vi "FPGA_small2-2.vi"() -> ()   [LabVIEW 2018]
uses:
  <vilib>/Platform/TimedLoop/XDataNode/timing_clust.ctl
  <vilib>/Platform/TimedLoop/XDataNode/nitl_modes.ctl
  <vilib>/Platform/TimedLoop/XDataNode/wakeup.ctl
  <vilib>/rvi/Emulation/niFpgaGetClockAttributes.vi
  <vilib>/rvi/Emulation/niFpgaSctlEmulationGetInTimedLoop.vi
  <vilib>/rvi/Emulation/niFpgaEmulationReportErrorSimple.vi
  <vilib>/rvi/eio/common/nirviEmuTemplateMethod_errors.vi
  <vilib>/rvi/Emulation/niFpgaCriticalErrorInLSC.vi
  <vilib>/rvi/Emulation/niFpgaProcessEmulError.vi
  <vilib>/eio/EIONode/EIONode.xnode
  <vilib>/platform/TimedLoop/XDataNode/XDataNode.xnode
  <vilib>/Platform/TimedLoop/XDataNode/XDNodeRunTimeDep.lvlib
panel:
  in  "speed_scale":i16=1500
  out "speed":i16
  in  "offtrack limit":i16=1500
  out "AI0":u16=1344
  out "dAI":i16=8
  in  "delay ai ms":u32=1
  in  "pwm_val":u32=100
  in  "dt_pwm_us":u32=30 caption="Count(uSec)"
  out "busy":bool
  in  "dt_ctrl_us":u32=1 caption="delay_M_ms"
  in  "set_point":i16
  in  "stop_band":i16=4
  in  "inv":bool=TRUE
  out "gap_pos":i16=-1
  out "backward":bool
  out "position":i16=1241
  out "err cnt":i16
  in  "reset":bool
  out "off_track":bool
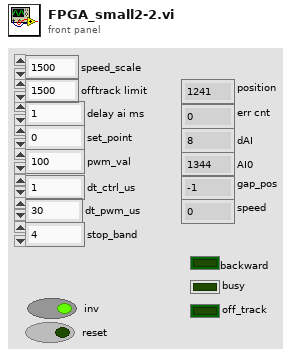
[diagram p1: front panel]
types:
  T1 = typedef "XDNodeRunTimeDep.lvlib/timing_clust.ctl" = cluster{"Expected End [f-1]":u64, "Actual End [f-1]":u64, "Finished Late? [f-1]":bool, "Expected End [i-1]":u64, "Actual End [i-1]":u64, "Finished Late? [i-1]":bool, "Expected Start [i]":u64, "Actual Start [i]":u64, "Expected Start [f]":u64, "Actual Start [f]":u64, "Source Name":string, "Structure Name":string, "Period":i64, "Deadline":i64, "Offset":i64, "Start":i64, "Priority":i32, "Timeout":i32, "Mode":T2, "Wakeup Reason":T3, "Error":errorcluster, "Source Type":string, "Secondary Source Type":string, "Global End Time":u64, "Global Start Time":u64, "Frame Duration":u64, "Iteration Duration":u64, "Assigned CPU":i32, "I/O Scan Engine Mode":u32}
  T2 = typedef "XDNodeRunTimeDep.lvlib/nitl_modes.ctl" = enum32{"No Change", "Process missed periods, maintain original phase", "Discard missed periods, maintain original phase", "Process missed periods, ignore original phase", "Discard missed periods, ignore original phase"}
  T3 = typedef "XDNodeRunTimeDep.lvlib/wakeup.ctl" = enum32{"Normal", "Aborted", "Asynchronous wakeup", "Timing source error", "Timed loop error", "Timeout"}
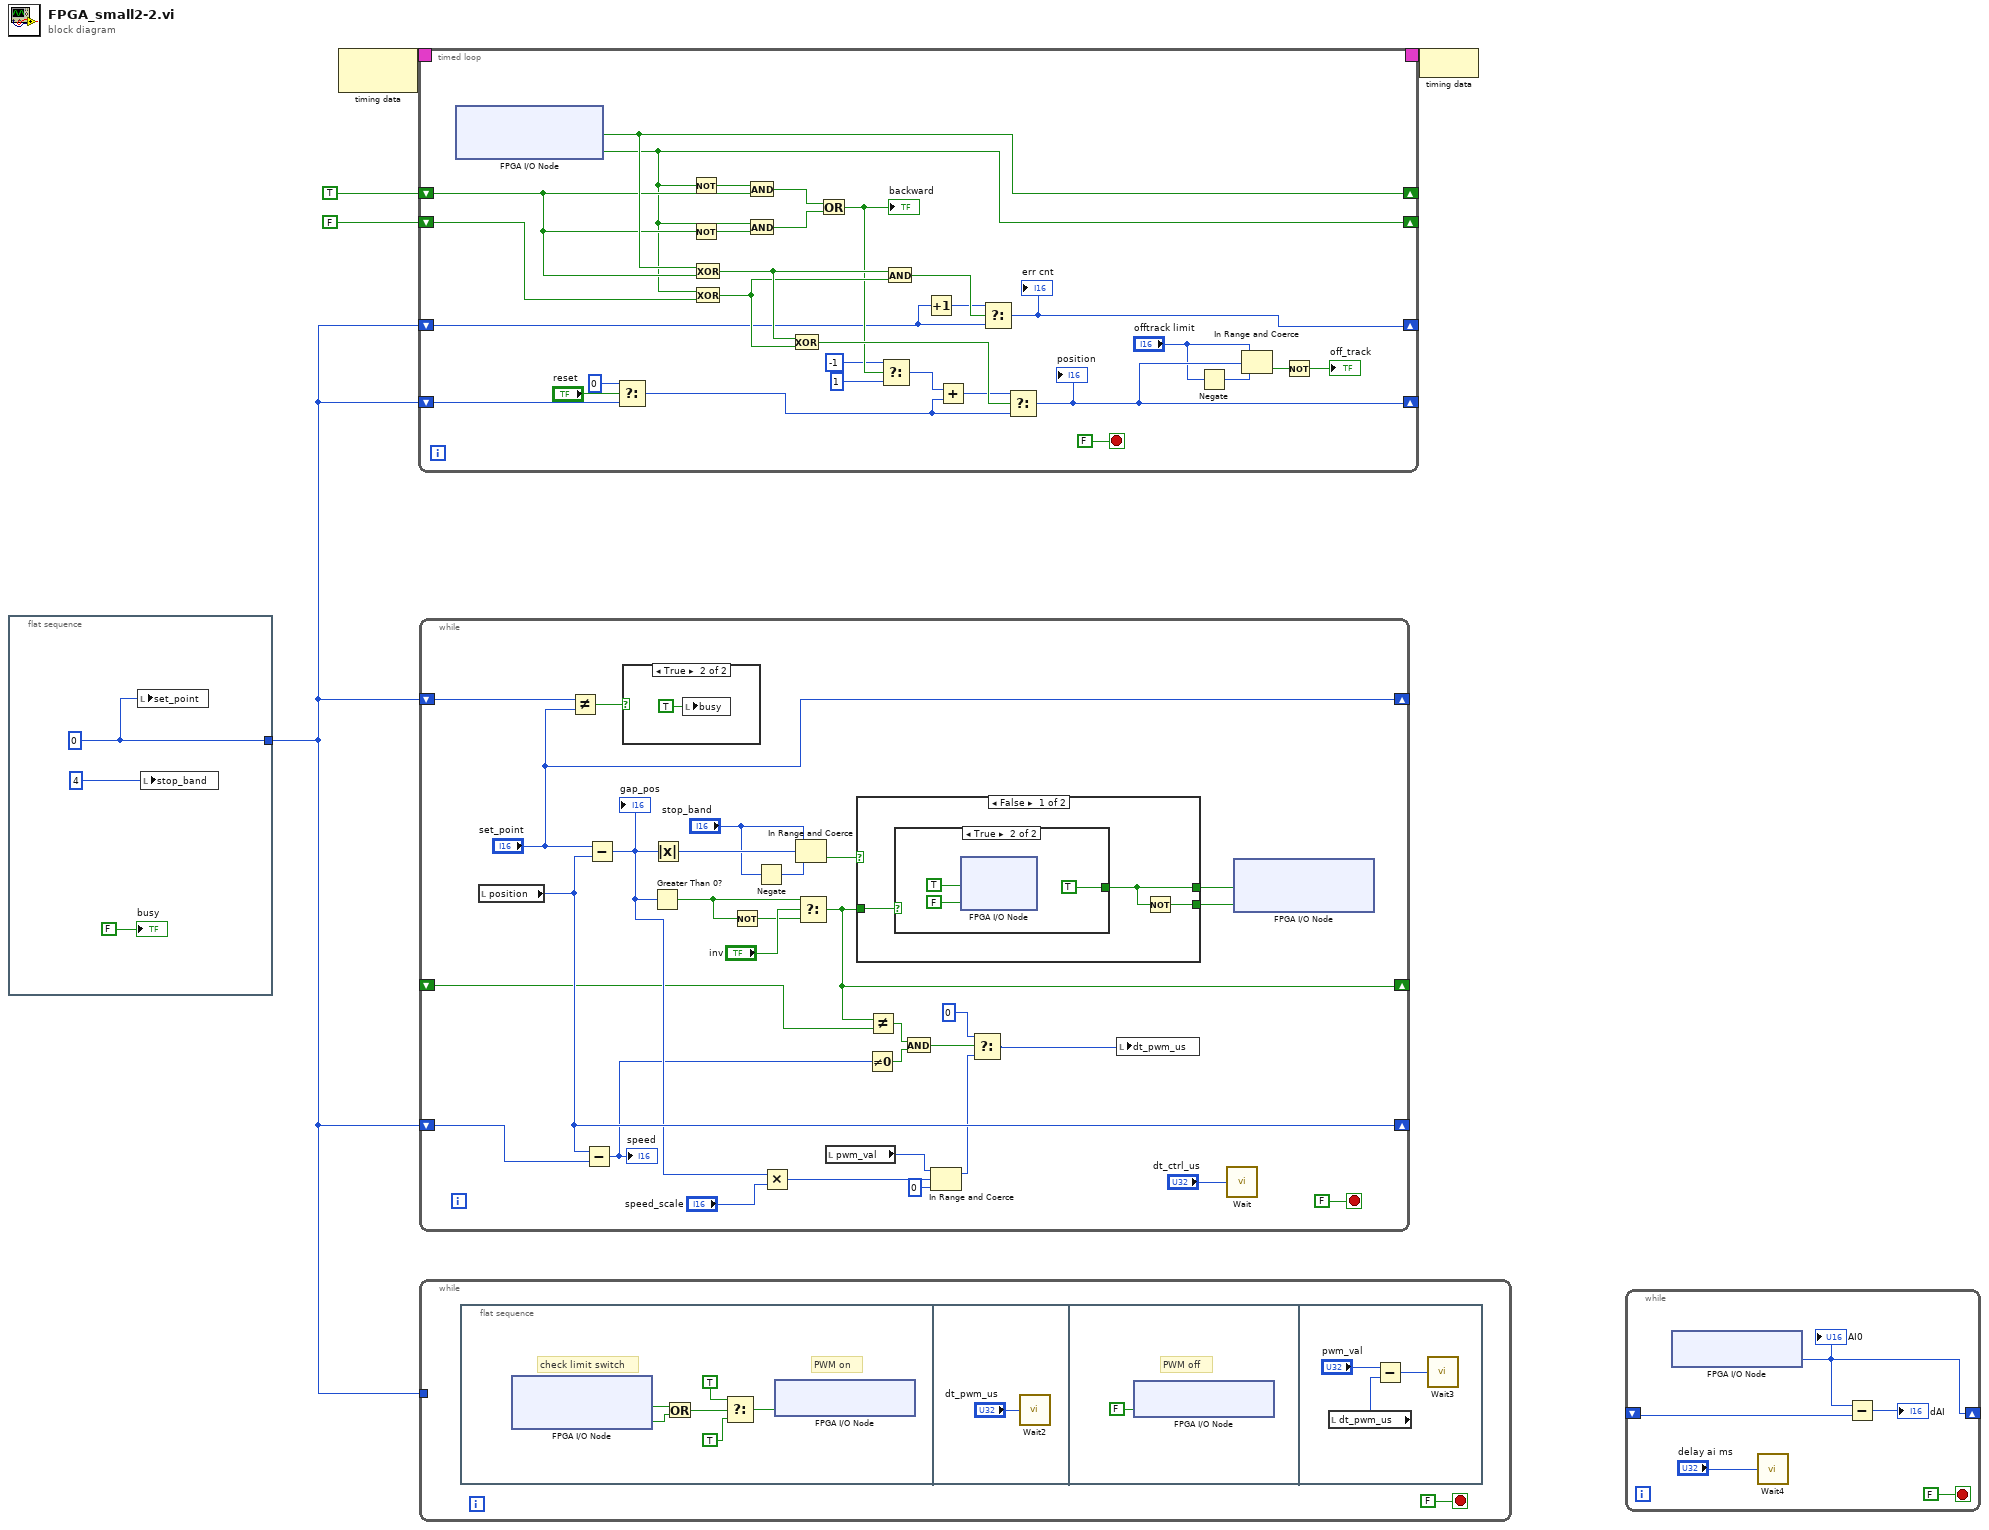
[diagram p0: block diagram]
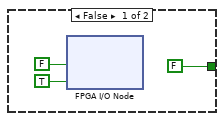
[diagram p3: hidden frame]
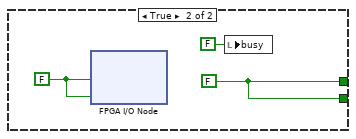
[diagram p4: hidden frame]
diagram:
  n1 = flat-sequence {
    tunnel: [w7] -> w1
    frame #0 {
      w7 = i16 0
      n2 = local write "set_point"(w7) -> ()
      n3 = local write "stop_band"(i16 4 ("dead band")) -> ()
      "busy" <- FALSE ("status")
    }
  }
  n4 = node-c288() -> (w5:T1)  [unwired: 1 in]
  n5 = timed-loop {
    timing: w5 -> [_]
    timing-out: [_] -> w4
    shift-right: [w33] -> _
    shift-left: TRUE ("ConnectorA/DIO11") -> [w32]
    shift-right: [w31] -> _
    shift-left: FALSE ("ConnectorA/DIO12") -> [w30]
    shift-right: [w13] -> _
    shift-left: w1 -> [w16]
    shift-right: [w18] -> _
    shift-left: w1 -> [w19]
    stop <- FALSE stop-if-true
    n6 = xnode "FPGA I/O Node"() -> ("ConnectorA/DIO11"=w33:bool, "ConnectorA/DIO12"=w31:bool)  [unwired: 2 in, 2 out]
    n7 = Select(t=i16 0, s="reset", f=w16) -> (s? t:f=w14:i16)
    n8 = Not(x=w31) -> (.not. x?=w37:bool)
    n9 = Not(x=w32) -> (.not. x?=w36:bool)
    n10 = Exclusive Or(1:w32, 2:w33) -> (0:w29:bool)
    n11 = Exclusive Or(1:w30, 2:w31) -> (0:w28:bool)
    n12 = And(x=w37, y=w32) -> (x .and. y?=w34:bool)
    n13 = And(x=w31, y=w36) -> (x .and. y?=w35:bool)
    n14 = Exclusive Or(1:w28, 2:w29) -> (0:w27:bool)
    n15 = Or(x=w34, y=w35) -> (x .or. y?=w26:bool)
    "backward" <- w26
    n16 = Select(t=i16 -1, s=w26, f=i16 1) -> (s? t:f=w23:i16)
    n17 = And(x=w29, y=w28) -> (x .and. y?=w21:bool)
    n18 = Increment(x=w19) -> (x+1=w20:i16)
    n19 = Add(x=w23, y=w14) -> (x+y=w22:i16)
    n20 = Select(t=w20, s=w21, f=w19) -> (s? t:f=w18:i16)
    "err cnt" <- w18
    n21 = Select(t=w22, s=w27, f=w14) -> (s? t:f=w13:i16)
    "position" <- w13
    n22 = Negate(x="offtrack limit") -> (-x=w10:i16)
    n23 = In Range and Coerce(upper limit="offtrack limit", x=w13, lower limit=w10) -> (In Range?=w12:bool)  [unwired: 1 out]
    n24 = Not(x=w12) -> (.not. x?=→"off_track":bool)
  }
  n25 = while {
    shift-right: ["set_point"] -> _
    shift-left: w1 -> [w58]
    shift-right: [w56] -> _
    shift-left: w1 -> [w55]
    shift-right: [w49] -> _
    shift-left: _ -> [w48]
    stop <- FALSE stop-if-true
    n26 = local read "position"() -> (w56:i16)
    n27 = Not Equal?(x=w58, y="set_point") -> (x != y?=w57:bool)
    n28 = Subtract(x=w56, y=w55) -> (x-y=w47:i16)
    "speed" <- w47
    n29 = Subtract(x="set_point", y=w56) -> (x-y=w53:i16)
    "gap_pos" <- w53
    n30 = case shown="True" w57 {
      frame False {
      }
      frame True {
        n31 = local write "busy"(TRUE ("busy")) -> ()
      }
    }
    n32 = Greater Than 0?(x=w53) -> (x > 0?=w60:bool)
    n33 = Absolute Value(x=w53) -> (abs(x)=w66:i16)
    n34 = Not(x=w60) -> (.not. x?=w61:bool)
    n35 = Negate(x="stop_band") -> (-x=w65:i16)
    n36 = Multiply(x=w53, y="speed_scale") -> (x*y=w52:i16)
    n37 = In Range and Coerce(upper limit="stop_band", x=w66, lower limit=w65) -> (In Range?=w63:bool)  [unwired: 1 out]
    n38 = Select(t=w60, s="inv", f=w61) -> (s? t:f=w49:bool)
    n39 = local read "pwm_val"() -> (w51:u32)
    n40 = case shown="False" w63 {
      tunnel: [w74 w83] -> w68
      tunnel: [w73 w83] -> w67
      tunnel: w49 -> [w72 _]
      frame False {
        n41 = case shown="True" w72 {
          tunnel: [FALSE ("dir") TRUE ("dir")] -> w73
          frame False {
            n42 = xnode "FPGA I/O Node"("LED0"=FALSE, "LED1"=TRUE) -> ()  [unwired: 2 in, 2 out]
          }
          frame True {
            n43 = xnode "FPGA I/O Node"("LED0"=TRUE, "LED1"=FALSE) -> ()  [unwired: 2 in, 2 out]
          }
        }
        n44 = Not(x=w73) -> (.not. x?=w74:bool)
      }
      frame True {
        w81 = FALSE ("LED0")
        w83 = FALSE ("dir")
        n45 = xnode "FPGA I/O Node"("LED0"=w81, "LED1"=w81) -> ()  [unwired: 2 in, 2 out]
        n46 = local write "busy"(FALSE ("busy")) -> ()
      }
    }
    n47 = Not Equal To 0?(x=w47) -> (x != 0?=w46:bool)
    n48 = Not Equal?(x=w49, y=w48) -> (x != y?=w45:bool)
    n49 = And(x=w45, y=w46) -> (x .and. y?=w44:bool)
    n50 = In Range and Coerce(upper limit=w51, x=w52, lower limit=u32 0) -> (coerced(x)=w42:u32)  [unwired: 1 out]
    n51 = Select(t=u32 0 ("lower limit"), s=w44, f=w42) -> (s? t:f=w41:u32)
    n52 = local write "dt_pwm_us"(w41) -> ()
    n53 = call "Wait"("Count(uSec)"="dt_ctrl_us") -> ()  [unwired: 1 out]
    n54 = xnode "FPGA I/O Node"("ConnectorA/DIO6"=w67, "ConnectorA/DIO5"=w68) -> ()  [unwired: 2 in, 2 out]
  }
  n55 = while {
    tunnel: w1 -> [_]
    stop <- FALSE stop-if-true
    n56 = flat-sequence {
      frame #0 {
        # "check limit switch"
        # "PWM on"
        n57 = xnode "FPGA I/O Node"() -> ("ConnectorA/DIO0"=w89:bool, "ConnectorA/DIO1"=w90:bool)  [unwired: 2 in, 2 out]
        n58 = Or(x=w89, y=w90) -> (x .or. y?=w88:bool)
        n59 = Select(t=TRUE, s=w88, f=TRUE ("ConnectorA/DIO8")) -> (s? t:f=w87:bool)
        n60 = xnode "FPGA I/O Node"("ConnectorA/DIO8"=w87) -> ()  [unwired: 1 in, 1 out]
      }
      frame #1 {
        n61 = call "Wait2"("Count(uSec)"="dt_pwm_us") -> ()  [unwired: 1 out]
      }
      frame #2 {
        # "PWM off"
        n62 = xnode "FPGA I/O Node"("ConnectorA/DIO8"=FALSE) -> ()  [unwired: 1 in, 1 out]
      }
      frame #3 {
        n63 = local read "dt_pwm_us"() -> (w95:u32)
        n64 = Subtract(x="pwm_val", y=w95) -> (x-y=w93:u32)
        n65 = call "Wait3"("Count(uSec)"=w93) -> ()  [unwired: 1 out]
      }
    }
  }
  n66 = node-c288(w4) -> ()
  n67 = while {
    shift-right: [w97] -> _
    shift-left: _ -> [w98]
    stop <- FALSE stop-if-true
    n68 = xnode "FPGA I/O Node"() -> ("ConnectorA/AI0"=w97:u16)  [unwired: 1 in, 1 out]
    "AI0" <- w97
    n69 = call "Wait4"("Count(mSec)"="delay ai ms") -> ()  [unwired: 1 out]
    n70 = Subtract(x=w97, y=w98) -> (x-y=→"dAI":u16)
  }
